vi "gfitsio-delete-current-hdu.vi"(8 "error in (no error)":errorcluster, 11 "gfits refnum":T1) -> (0 "error out":errorcluster, 3 "dup gfits refnum":T1)   [LabVIEW 2011, in "gfitsio.lvlib"]
doc: "Delete the current HDU (CHDU) in the FITS file. Any following HDUs will be shifted forward in the file, to fill in the gap created by the deleted HDU. In the case of deleting the primary array (the first HDU in the file) then the current primary array will be replace by a null primary array containing the minimum set of required keywords and no data. If there are more extensions in the file following the one that is deleted, then the the CHDU will be redefined to point to the following extension. If there are no following extensions then the CHDU will be redefined to point to the previous HDU."
uses:
  gfitsio.lvlib
  gfitsio-refnum.ctl
  gfitsio.dll
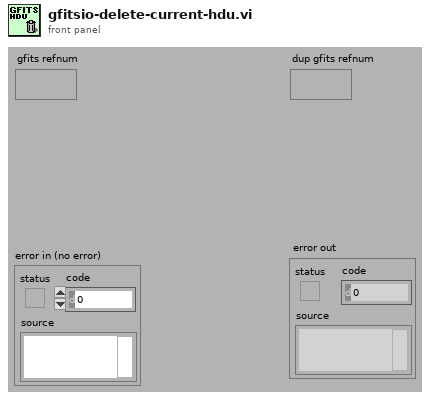
[diagram p1: front panel]
types:
  T1 = typedef "gfitsio.lvlib/gfitsio-refnum.ctl" = refnum<k1>
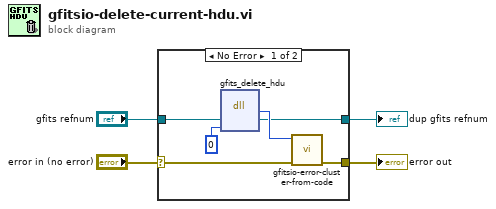
[diagram p0: block diagram]
diagram:
  n1 = case shown="No Error" "error in (no error)" {
    selector: "error in (no error)" -> [w8 w12]
    tunnel: [w10 w12] -> w4
    tunnel: "gfits refnum" -> [w6 w11]
    tunnel: [w7 w11] -> w2
    frame No Error {
      n2 = dll-call lib="C:/jul 1 BonOmm 2.0/SubVIs/gfitsio/gfitsio.dll" fn="gfits_delete_hdu"("gfits refnum"=w6, "tbltype"=0) -> (w9:i32, "gfits refnum"=w7:T1)  [unwired: 4 in, 2 out]
      n3 = call "gfitsio-error-cluster-from-code.vi"("error in (no error)"=w8, "error code"=w9) -> ("error out"=w10:errorcluster)  [unwired: 9 in]
    }
    frame Error {
    }
  }
  "error out" <- w4
  "dup gfits refnum" <- w2
